vi "Dodanie wskazanego punktu z listy współrzędnych do mapy 2 optymalizowane.vi"(0 "Mapa terenu":picture, 1 "Rozmiar mapy":T1={"left"=0, "top"=0, "right"=836, "bottom"=597}, 5 "Długość piksela w metrach":dbl, 9 "Nr punktu":i16, 11 "Lista współrzędnych":string[][](array[string]), 12 "Właściwości punktów z listy":T2) -> (4 "Mapa z wprowadzonym punktem":picture)   [LabVIEW 2015]
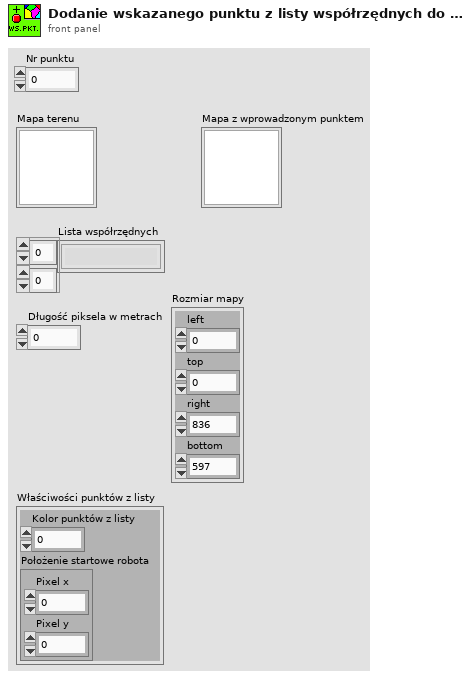
[diagram p1: front panel]
types:
  T1 = cluster{"left":i16, "top":i16, "right":i16, "bottom":i16}
  T2 = cluster{"Kolor punktów z listy":u32, "Położenie startowe robota":cluster{"Pixel x":i16, "Pixel y":i16}}
  T3 = cluster{"Width":u16, "Style":enum32{"Solid", "Dash", "Dot", "DashDot", "DashDotDot"}}
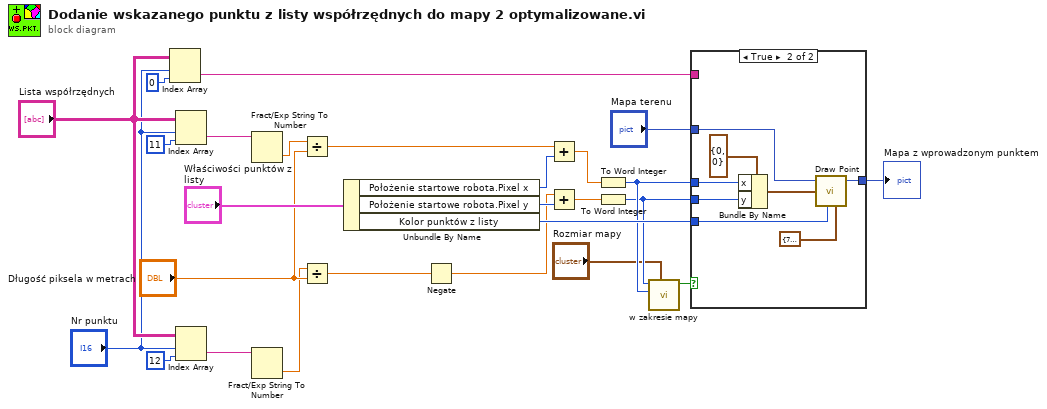
[diagram p0: block diagram]
diagram:
  n1 = Index Array(array="Lista współrzędnych", index (row)="Nr punktu", index (col)=0 ("disabled index (col)")) -> (element=w18:string)
  n2 = Index Array(array="Lista współrzędnych", index (row)="Nr punktu", index (col)=11 ("disabled index (col)")) -> (element=w13:string)
  n3 = Index Array(array="Lista współrzędnych", index (row)="Nr punktu", index (col)=12 ("disabled index (col)")) -> (element=w17:string)
  n4 = Fract/Exp String To Number(string=w13) -> (number=w19:dbl)  [unwired: 3 in, 1 out]
  n5 = Fract/Exp String To Number(string=w17) -> (number=w21:dbl)  [unwired: 3 in, 1 out]
  n6 = Divide(x=w19, y="Długość piksela w metrach") -> (x/y=w7:dbl)
  n7 = Divide(x=w21, y="Długość piksela w metrach") -> (x/y=w6:dbl)
  n8 = Unbundle By Name("Właściwości punktów z listy") -> ("Położenie startowe robota.Pixel x"=w23:i16, "Położenie startowe robota.Pixel y"=w24:i16, "Kolor punktów z listy"=w25:u32)
  n9 = Negate(x=w6) -> (-x=w20:dbl)
  n10 = Add(x=w7, y=w23) -> (x+y=w9:dbl)
  n11 = Add(x=w20, y=w24) -> (x+y=w8:dbl)
  n12 = To Word Integer(number=w9) -> (16bit integer=w5:i16)
  n13 = To Word Integer(number=w8) -> (16bit integer=w4:i16)
  n14 = call "w zakresie mapy.vi"("Rozmiar mapy"="Rozmiar mapy", "Pixel x"=w5, "Pixel y"=w4) -> ("Boolean"=w3:bool)  [unwired: 8 in]
  n15 = case shown="True" w3 {
    tunnel: w25 -> [_ w28]
    tunnel: w18 -> [_ _]
    tunnel: [w27 w34] -> w14
    tunnel: "Mapa terenu" -> [w27 w35]
    tunnel: w4 -> [_ w29]
    tunnel: w5 -> [_ w30]
    frame False {
    }
    frame True {
      n16 = Bundle By Name(cluster=cluster{"x":i16, "y":i16} {"x"=0, "y"=0} ("point(x,y)"), "x"=w30, "y"=w29) -> (w31:cluster{"x":i16, "y":i16})
      n17 = call <vilib>:"Draw Point.vi"("picture"=w35, "point(x,y)"=w31, "color(black)"=w28, "pen"=T3 {"Width"=7, "Style"=enum."Solid"}) -> ("new picture"=w34:picture)  [unwired: 5 in]
    }
  }
  "Mapa z wprowadzonym punktem" <- w14
